vi "__test.vi"() -> ()   [LabVIEW 2011]
uses:
  lua_State.ctl
panel:
  in  "lua_State *luaL_newstate":T1
  out "数值":u64
  out "const char *lua_pushstring":string
  out "lua_type":i32(ring) items=["LUA_TNONE"=-1, "LUA_TNIL"=0, "LUA_TBOOLEAN"=1, "LUA_TLIGHTUSERDATA"=2, "LUA_TNUMBER "=3, "LUA_TSTRING"=4, "LUA_TTABLE"=5, "LUA_TFUNCTION"=6, "LUA_TUSERDATA"=7, "LUA_TTHREAD"=8, "LUA_NUMTAGS "=9]
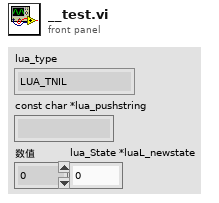
[diagram p1: front panel]
types:
  T1 = typedef "lua_State.ctl" = u64
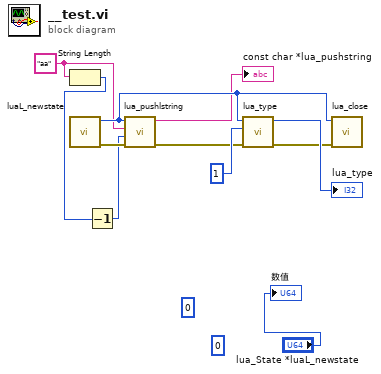
[diagram p0: block diagram]
diagram:
  (unwired) T1 0 ("lua_State *luaL_newstate")
  (unwired) T1 0 ("lua_State *luaL_newstate")
  w4 = "aa" ("const char *s")
  n1 = String Length(string=w4) -> (length=w3:i32)
  n2 = call "luaL_newstate.vi"() -> ("error out"=w7:errorcluster, "lua_State *luaL_newstate"=w8:u64)  [unwired: 10 in]
  n3 = Decrement(x=w3) -> (x-1=w2:i32)
  n4 = call "lua_pushlstring.vi"("error in"=w7, "size_t len"=w2, "const char *s"=w4, "lua_State *L"=w8) -> ("error out"=w5:errorcluster, "const char *lua_pushlstring"=→"const char *lua_pushstring":string)  [unwired: 6 in]
  n5 = call "lua_type.vi"("error in"=w5, "int index"=1, "lua_State *L"=w8) -> ("error out"=w9:errorcluster, "lua_type"=→"lua_type":i32)  [unwired: 7 in]
  n6 = call "lua_close.vi"("error in"=w9, "lua_State *L"=w8) -> ()  [unwired: 9 in, 1 out]
  "数值" <- "lua_State *luaL_newstate"
